vi "rolling_number.vi"(4 "Position":cluster{"left":i16, "top":i16}={"left"=30, "top"=5}, 5 "Background color":u32(colorbox)=14803425, 7 "number":dbl=123.0, 10 "pict in":picture) -> (3 "pict out":picture)   [LabVIEW 2011]
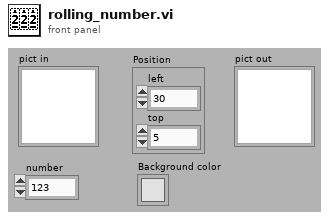
[diagram p1: front panel]
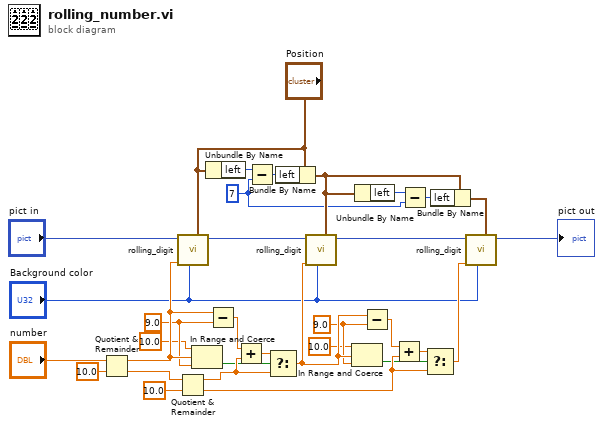
[diagram p0: block diagram]
diagram:
  w22 = 9.0 ("lower limit")
  w1 = i16 7 ("y")
  w11 = 9.0 ("lower limit")
  n1 = Quotient & Remainder(x="number", y=10.0) -> (x-y*floor(x/y)=w26:dbl, floor(x/y)=w28:dbl)
  n2 = call "rolling_digit.vi"("Position"="Position", "Background color"="Background color", "value"=w26, "pict in"="pict in") -> ("pict out"=w18:picture)  [unwired: 6 in]
  n3 = Quotient & Remainder(x=w28, y=10.0) -> (x-y*floor(x/y)=w29:dbl, floor(x/y)=w32:dbl)
  n4 = In Range and Coerce(upper limit=10.0, x=w26, lower limit=w11) -> (In Range?=w10:bool)  [unwired: 1 out]
  n5 = Unbundle By Name("Position") -> ("left"=w14:i16)
  n6 = Subtract(x=w26, y=w11) -> (x-y=w12:dbl)
  n7 = Add(x=w12, y=w29) -> (x+y=w13:dbl)
  n8 = Subtract(x=w14, y=w1) -> (x-y=w15:i16)
  n9 = Select(t=w13, s=w10, f=w29) -> (s? t:f=w31:dbl)
  n10 = Bundle By Name(cluster="Position", "left"=w15) -> (w16:cluster{"left":i16, "top":i16})
  n11 = call "rolling_digit.vi"("Position"=w16, "Background color"="Background color", "value"=w31, "pict in"=w18) -> ("pict out"=w3:picture)  [unwired: 6 in]
  n12 = In Range and Coerce(upper limit=10.0, x=w31, lower limit=w22) -> (In Range?=w25:bool)  [unwired: 1 out]
  n13 = Unbundle By Name(w16) -> ("left"=w6:i16)
  n14 = Subtract(x=w31, y=w22) -> (x-y=w23:dbl)
  n15 = Add(x=w23, y=w32) -> (x+y=w24:dbl)
  n16 = Subtract(x=w6, y=w1) -> (x-y=w5:i16)
  n17 = Select(t=w24, s=w25, f=w32) -> (s? t:f=w27:dbl)
  n18 = Bundle By Name(cluster=w16, "left"=w5) -> (w7:cluster{"left":i16, "top":i16})
  n19 = call "rolling_digit.vi"("Position"=w7, "Background color"="Background color", "value"=w27, "pict in"=w3) -> ("pict out"=→"pict out":picture)  [unwired: 6 in]
